vi "Create All Message Queues.vi"(8 "error in (no error)":errorcluster, 11 "This VI":refnum<vi>) -> (0 "error out":errorcluster, 3 "Message Queues out":T1)   [LabVIEW 2024, in "MCU_Flashing.lvlib" / "MCU Message Queue.lvlib"]
doc: "This VI creates and initializes all the message queues for your application. If your application requires more than one message queue, right-click the \"Message Queues\" constant above and select Open Type Def. Add the new Message Queue(s) to the type definition, then initialize them in this VI."
uses:
  MCU Message Queue.lvlib
  All Message Queues.ctl
  Enqueue Message (Single).vi
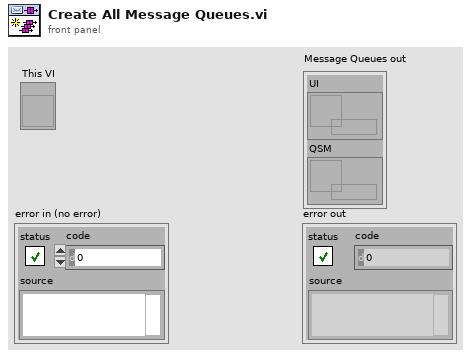
[diagram p1: front panel]
types:
  T1 = typedef "MCU_Flashing.lvlib/MCU Message Queue.lvlib/All Message Queues.ctl" = cluster{"UI":refnum<queue>, "QSM":refnum<queue>}
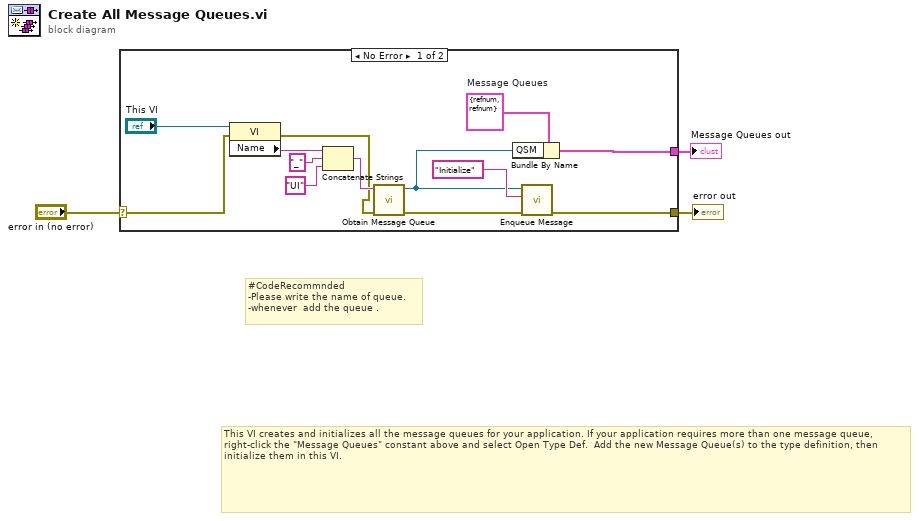
[diagram p0: block diagram]
diagram:
  # "#CodeRecommnded\n-Please write the name of queue.\n-whenever  add the queue ."
  # "This VI creates and initializes all the message queues for your application. If your application requires more than one message queue, right-click the \"Message Queues\" constant above and select Open Type Def.  Add the new Message Queue(s) to the type definition, then initialize them in this VI."
  n1 = case shown="No Error" "error in (no error)" {
    selector: "error in (no error)" -> [w5 w17]
    tunnel: [w16 w17] -> w3
    tunnel: [w14 _] -> w2
    frame No Error {
      w15 = T1 {"UI"=refnum, "QSM"=refnum}  # Message Queues
      n2 = property class="VI"(reference="This VI", error in=w5) -> (error out=w4:errorcluster, "Name"=w10:string)  [unwired: 1 out]
      n3 = Concatenate Strings(w10, "_" ("string"), "UI" ("string")) -> (w9:string)
      n4 = call "Obtain Message Queue.vi"("error in (no error)"=w4, "Queue Name"=w9) -> ("error out"=w13:errorcluster, "Message Queue"=w11:refnum<queue>)  [unwired: 8 in]
      n5 = Bundle By Name(cluster=w15, "QSM"=w11) -> (w14:T1)
      n6 = call-poly "Enqueue Message.vi"("error in (no error)"=w13, "Message"="Initialize", "Message Queue"=w11) -> ("error out"=w16:errorcluster)  [unwired: 7 in, 1 out]
    }
    frame Error {
    }
  }
  "Message Queues out" <- w2
  "error out" <- w3
